vi "Drive Encoder Get.vi"(10 "AIDeviceRef Left":T1={"DevStatus"={"status"=FALSE, "code"=0, "source"=""}, "Analog Channel"=enum."AI 1"}, 11 "AIDeviceRef Right":T1={"DevStatus"={"status"=FALSE, "code"=0, "source"=""}, "Analog Channel"=enum."AI 1"}) -> ()   [LabVIEW 2015]
uses:
  <vilib>/Rock Robotics/WPI/AnalogChannel/WPI_AnalogChannelDevRef.ctl
  <vilib>/Rock Robotics/SystemInterfaces/AI/FPGA_AIChannel.ctl
  Robot Values.vi
  <vilib>/ptbypt/NI_PtbyPt.lvlib
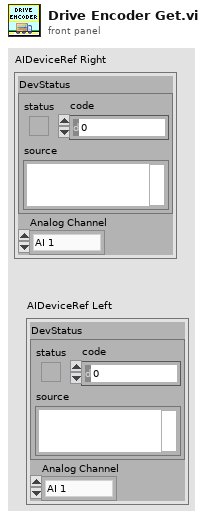
[diagram p1: front panel]
types:
  T1 = typedef "WPI_AnalogChannelDevRef.ctl" = cluster{"DevStatus":errorcluster, "Analog Channel":T2}
  T2 = typedef "FPGA_AIChannel.ctl" = enum8{"AI 0", "AI 1", "AI 2", "AI 3", "AI MXP 0", "AI MXP 1", "AI MXP 2", "AI MXP 3", "Invalid"}
  T3 = cluster{"Tracking Tote?":bool, "ToteRightSpeed":dbl, "ToteLeftSpeed":dbl, "Drive Encoder reset":bool, "Right Wheel \n(Cm)":dbl, "Left Wheel \n(Cm)":dbl}
  T4 = cluster{"Lift Encoder Height Right (cm)":dbl, "Lift Encoder Height Left (cm)":dbl, "Right Prox":bool, "Left Prox":bool, "Gyro Angle":dbl, "Gyro anglar rate":dbl, "Gyro Reset":bool, "Drive encoder Dash reset":bool}
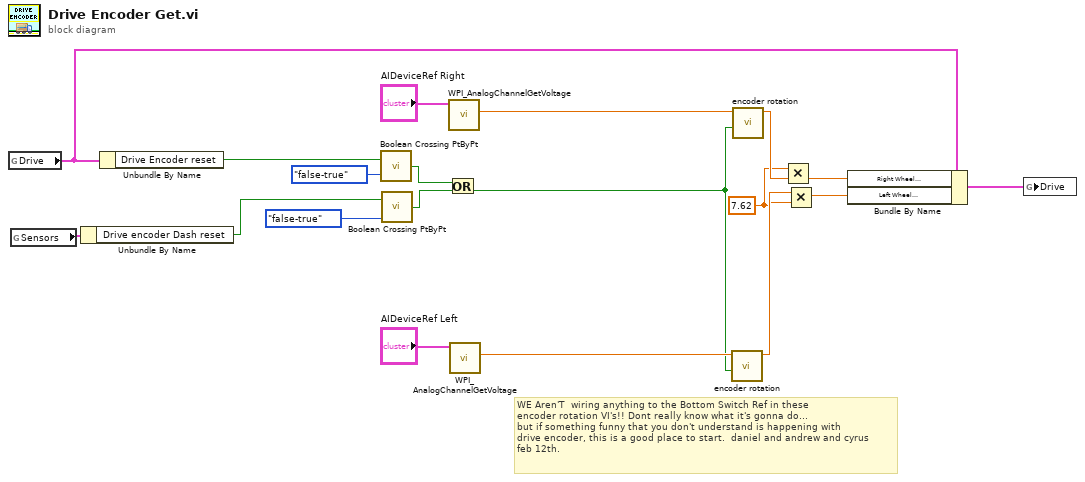
[diagram p0: block diagram]
diagram:
  w9 = 7.62 ("y")
  # "WE Aren'T  wiring anything to the Bottom Switch Ref in these \nencoder rotation VI's!! Dont really know what it's gonna do...\nbut if something funny that you don't understand is happening with\ndrive encoder, this is a good place to start.  daniel and andrew and cyrus\nfeb 12th."
  n1 = global read "Robot Values.vi" "Drive"() -> (w18:T3)
  n2 = global read "Robot Values.vi" "Sensors"() -> (w2:T4)
  n3 = Unbundle By Name(w2) -> ("Drive encoder Dash reset"=w1:bool)
  n4 = Unbundle By Name(w18) -> ("Drive Encoder reset"=w7:bool)
  n5 = call <vilib>:"Boolean Crossing PtByPt.vi"("direction"=enum16{"either", "false-true", "true-false"}."false-true", "input"=w7) -> ("crossing"=w4:bool)  [unwired: 1 in]
  n6 = call <vilib>:"Boolean Crossing PtByPt.vi"("direction"=enum16{"either", "false-true", "true-false"}."false-true", "input"=w1) -> ("crossing"=w3:bool)  [unwired: 1 in]
  n7 = Or(x=w4, y=w3) -> (x .or. y?=w5:bool)
  n8 = call <vilib>:"WPI_AnalogChannelGetVoltage.vi"("AIDeviceRef"="AIDeviceRef Right") -> ("Voltage"=w14:dbl)  [unwired: 8 in, 2 out]
  n9 = call <vilib>:"WPI_AnalogChannelGetVoltage.vi"("AIDeviceRef"="AIDeviceRef Left") -> ("Voltage"=w12:dbl)  [unwired: 8 in, 2 out]
  n10 = call "encoder rotation.vi"("Reset Encoder"=w5, "Voltage"=w12) -> ("Angle(rad)"=w16:dbl)  [unwired: 7 in, 2 out]
  n11 = call "encoder rotation.vi"("Reset Encoder"=w5, "Voltage"=w14) -> ("Angle(rad)"=w17:dbl)  [unwired: 7 in, 2 out]
  n12 = Multiply(x=w9, y=w17) -> (x*y=w10:dbl)
  n13 = Multiply(x=w16, y=w9) -> (x*y=w11:dbl)
  n14 = Bundle By Name(cluster=w18, "Right Wheel \n(Cm)"=w10, "Left Wheel \n(Cm)"=w11) -> (w19:T3)
  n15 = global write "Robot Values.vi" "Drive"(w19) -> ()
